vi "Obtain Actual Voltage.vi"(8 "error in (no error)":errorcluster, 10 "Error Percentage":dbl format="%#_13g", 11 "DAC in":refnum<class "DAC.lvclass">) -> (0 "error out":errorcluster, 3 "DAC out":refnum<class "DAC.lvclass">)   [LabVIEW 2023, in "DAC.lvclass"]
uses:
  DAC.lvclass
  C:/Users/Ancy.Augustin/Downloads/INL DNL/INL DNL/Classes/Mode/Mode.lvclass
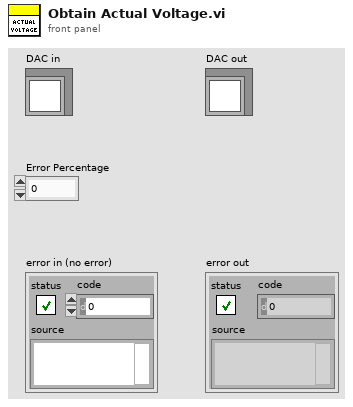
[diagram p1: front panel]
types:
  T1 = typedef "Transfer Function.ctl" = cluster{"Ideal voltage":dbl[], "Digital Code":dbl[]}
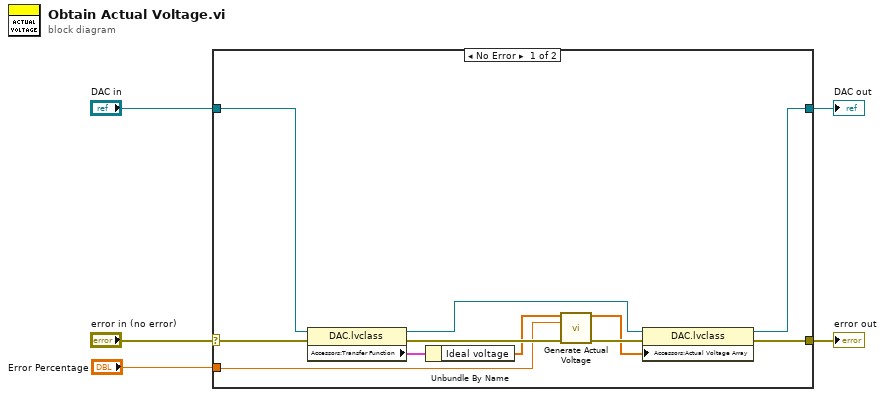
[diagram p0: block diagram]
diagram:
  n1 = case shown="No Error" "error in (no error)" {
    selector: "error in (no error)" -> [w16 w18]
    tunnel: [w9 w18] -> w4
    tunnel: [w6 w17] -> w2
    tunnel: "DAC in" -> [w13 w17]
    tunnel: "Error Percentage" -> [w10 _]
    frame No Error {
      n2 = property class="DAC.lvclass"(reference=w13, error in=w16) -> (reference out=w8:refnum<class "DAC.lvclass">, error out=w14:errorcluster, "Accessors:Transfer Function"=w12:T1)
      n3 = Unbundle By Name(w12) -> ("Ideal voltage"=w11:dbl[])
      n4 = call "Generate Actual Voltage.vi"("VoltageArray"=w11, "ErrorValue"=w10, "error in"=w14) -> ("ActualVoltageArray"=w7:dbl[], "error out"=w15:errorcluster)  [unwired: 11 in]
      n5 = property class="DAC.lvclass"(reference=w8, error in=w15, "Accessors:Actual Voltage Array"=w7) -> (reference out=w6:refnum<class "DAC.lvclass">, error out=w9:errorcluster)
    }
    frame Error {
    }
  }
  "error out" <- w4
  "DAC out" <- w2
